vi "NewMainImageRef.vi"(8 "error in (no error)":errorcluster, 11 "GenericCamera in":refnum<class "GenericCamera.lvclass">) -> (0 "error out":errorcluster, 3 "GenericCamera out":refnum<class "GenericCamera.lvclass">)   [LabVIEW 2013, in "GenericCamera.lvclass"]
uses:
  GenericCamera.lvclass
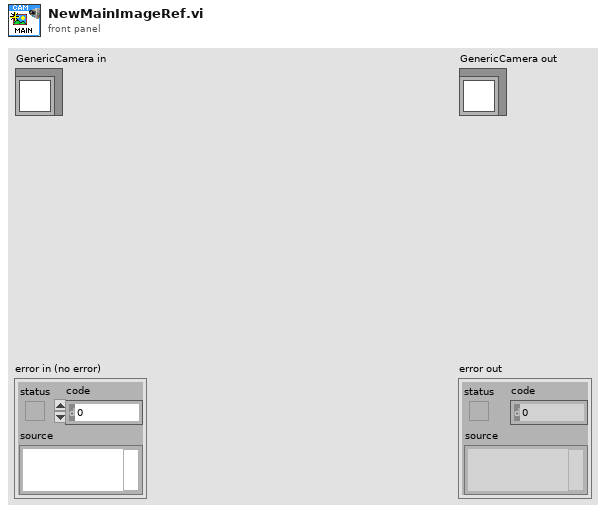
[diagram p1: front panel]
types:
  T1 = typedef "IMAQ Image.ctl" = refnum<image>
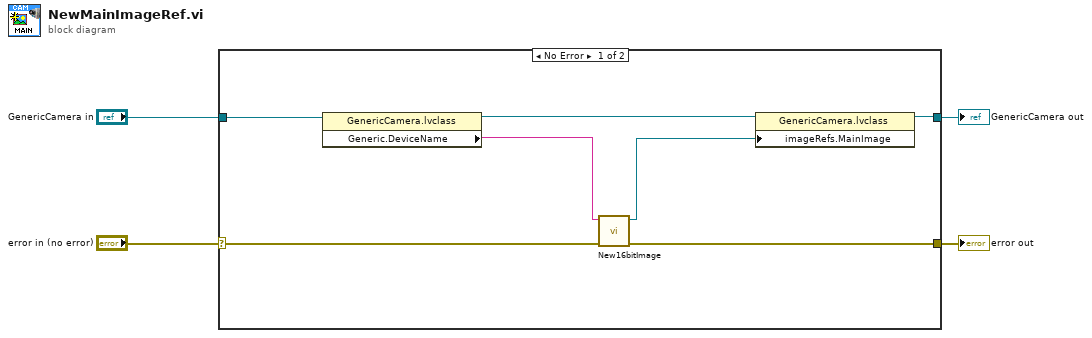
[diagram p0: block diagram]
diagram:
  n1 = case shown="No Error" "error in (no error)" {
    selector: "error in (no error)" -> [w9 w13]
    tunnel: [w7 w13] -> w3
    tunnel: [w6 w12] -> w1
    tunnel: "GenericCamera in" -> [w8 w12]
    frame No Error {
      n2 = property class="GenericCamera.lvclass"(reference=w8) -> (reference out=w11:refnum<class "GenericCamera.lvclass">, "Generic.DeviceName"=w5:string)  [unwired: 1 in, 1 out]
      n3 = call "New16bitImage.vi"("error in (no error)"=w9, "ImageName"=w5) -> ("error out"=w7:errorcluster, "Refnum out"=w10:T1)  [unwired: 8 in]
      n4 = property class="GenericCamera.lvclass"(reference=w11, "imageRefs.MainImage"=w10) -> (reference out=w6:refnum<class "GenericCamera.lvclass">)  [unwired: 1 in, 1 out]
    }
    frame Error {
    }
  }
  "error out" <- w3
  "GenericCamera out" <- w1
